vi "Big_LED_control.vi"() -> ()   [LabVIEW 2018]
uses:
  AT lib/AmateurStepperMotor.dll
  <instrlib>/niDMM/nidmm.llb/niDMM Function.ctl
  <instrlib>/niDMM/nidmm.llb/niDMM Resolution in Digits.ctl
  <instrlib>/niDCPower/nidcpower.llb/niDCPower Measurement Type.ctl
  <vilib>/Instr/_visa.llb/VISA Configure Serial Port (Instr).vi
  <instrlib>/niDMM/nidmm.llb/niDMM Configure Measurement Digits.vi
panel:
  in  "Tab Control 2":enum32{"Шаговик и офир", "Служебная область"}(tab)
  in  "milliseconds to wait":u32=1000
  in  "Go To":dbl
  out "Ophir 1 Char":dbl(graph)=7.0
  in  "DecelerationTime, s":dbl
  in  "AccelerationTime, s":dbl
  in  "HoldOn":bool
  in  "Ophir 1 units":string(combo)="1000" caption="Units"
  out "Ophir 1 Over Range":bool caption="Over Range"
  out "Ophir 1 Optical Power":dbl=7.0 caption="Power" format="%#_4g"
  out "Ophir 1 MAX":dbl=7.0200000000000005 caption="MAX" format="%#_5g"
  in  "Ophir 1 Clear":bool caption="Clear"
  in  "StepMultiplicationFactor":dbl=1.0
  in  "StepDivisor":i32(ring)=8 items=["D1"=1, "D2"=2, "D4"=4, "D8"=8, "D16"=16, "D32"=32]
  in  "Speed":dbl=1000.0
  in  "Погнали!":bool
  in  "Стоп GoTo":bool
  out "Готово":bool
  out "Position":dbl
  in  "Ophir 1 Info":u16(ring)=1 caption="Info" items=["Device : JUNO; s/n:903793", "Head : PD300R-3W   ; s/n:779628"]
  in  "new pos":dbl
  in  "set pos":bool
  out "Device Response":string="*\n"
  in  "Ophir 1 usb channel":i16 caption="usb channel"
  out "Ophir 1 dup Visa Session":refnum<visa-resource-name>="USB0::0x0BD3::0x0777::NI-VISA-60004::RAW" caption="dup Visa Session"
  in  "Ophir 1 Baud Rate (3:9600)":i16(ring)=3 caption="Baud Rate (3:9600)" items=["300", "1200", "4800", "9600", "19200", "38400"]
  out "Ophir 1 Real Optical Power":dbl=0.007 format="%.6e"
  in  "Ophir 1 GPIB Address (10)":string="10" caption="GPIB Address (10)"
  in  "Ophir 1 Port Number (default 2)":i16=1 caption="Port Number (default 2)" min=0 max=20
  in  "Ophir 1 Select Communication Protocol":u16(ring) caption="Select Communication Protocol" items=["USB", "RS232", "GPIB"]
  out "Ophir 1 error out":errorcluster caption="error out"
  in  "Ophir 1 error in (no error)":errorcluster caption="error in (no error)"
  in  "Ophir 1 Wait":u32=100 caption="Wait"
  out "IsOpen":bool=TRUE
  out "Ophir 1 Initialization":bool=TRUE caption="Initialization"
  in  "Tab Control":T1(tab)
  in  "POWER":bool
  in  "Стоп":bool
  in  "Resource Name":refnum<k15>="PXI1Slot2" caption="Источник питания"
  in  "Амперметр":refnum<k15>="PXI1Slot4" caption="NI DMM 1"
  in  "V_MB, V":dbl=5.0 caption="voltage level" format="%_6p"
  in  "curlim_V_MB, A":dbl=0.3 caption="current limit" format="%_6p"
  out "curmes_V_MB, A":dbl caption="measurement" format="%_6g"
  out "chart_0":dbl(graph)=-0.001986406197333734 caption="Waveform Chart 5"
  in  "voltlim_I_LED, V":dbl=2.0 caption="current limit" min=0.01 format="%_6p"
  in  "I_LED, A":dbl=0.005 caption="voltage level" format="%_6p"
  out "chart_1":dbl(graph) caption="Waveform Chart 5"
  out "voltmes_I_LED, V":dbl caption="measurement" format="%_6g"
  out "Current Char":dbl(graph)=0.0019995495676994324
  in  "Arduino":refnum<visa-resource-name>="COM14"
  in  "Сегменты":bool[](array[boolean])=[FALSE, FALSE, FALSE, FALSE, FALSE, FALSE, FALSE, FALSE, FALSE, FALSE, FALSE, FALSE, FALSE, FALSE, FALSE, FALSE, FALSE, FALSE]
  in  "Вольтметр":refnum<k15>="PXI1Slot5" caption="NI DMM 1"
  out "Voltage Char":dbl(graph)=nan
  in  "Port Name":string="COM7" caption="Порт шаговика"
  in  "wave_lenght":string="600"
  in  "Промер":bool caption="Промер сегмента"
  in  "NI DMM 1 Voltage Range 4":string(combo)="-1" caption="Range"
  in  "NI DMM 1 units 4":string(combo)="1" caption="Units"
  out "Voltage":dbl=nan format="%_6g"
  in  "NI DMM 1 Current Range 3":string(combo)="1" caption="Range"
  in  "NI DMM 1 units 3":string(combo)="1000" caption="Units"
  out "Current":dbl=0.0019995495676994324 format="%_6g"
  out "Разряд":dbl
  out "+/-":bool
  out "Power off":bool=TRUE
  in  "Command":string="Anode"
  in  "Записать":bool
  out "measure output file refnum":refnum<file>
  out "Voltage, V":dbl=nan caption="Measurement" format="%.5f"
  out "Current, A":dbl=1.9995495676994324e-06 caption="Measurement" format="%.5f"
  out "Тип индикатора":string="Anode"
  out "chart_2":dbl(graph)=4.286668577189643e-07
  in  "V_RES, V":dbl caption="voltage level" format="%_6p"
  out "curmes_V_RES, A":dbl caption="measurement" format="%_6g"
  in  "curlim_V_RES, A":dbl=0.1 caption="current limit" min=0.01 format="%_6p"
  in  "measure path":path=path "D:/NI LabVIEW/MultiOpto/MultiOpto_1.2/Logs/SEL"
  out "Enum":enum16{"Exit", "4", "Промер", "2", "1"}(ring)
  out "№ об-ца":dbl=-1.0
  out "Темп-ра":dbl=-1.0
  out "Сегмент":string
  # "Шаговик"
  # "Офир"
  # "Шаговик"
  # "Офир"
  # "position - это значение абсолютное"
  # "j"
  # "c"
  # "d"
  # "e"
  # "g"
  # "h"
  # "a"
  # "b"
  # "f"
  # "k"
  # "L"
  # "m"
  # "n"
  # "p"
  # "dp"
  # "all"
  # "V_MB 5 В\nогрничение 300 м\n\nV_LED 2,1 В\nограничение 200 м"
  # "единицы мА\nrange 1 А"
  # "1. каждый сегмент включаем по отдельности, резистором постраиваем ток до 10 мА\n2. напряжение V_LED при этом не меняется\n3. в такоом положении промеряем сегменты по отдельности\n4. для промера всего индикатора сразу подстраиваем напряжение при неизменном положении резисторов\n5. ток всех индикаторов = ток одного сегмента (10 мА) * число сегментов (15)\n6. добиваемся этого увеличением V_LED"
  # "единицы В\nrange AUTO"
  # "регклировка суммарного тока через индикатор"
  # "24.063\n\n     I          U\n20 мА  1.3 В\n20 мА  1.4 В\n 7 мА   1.15 В"
  # "24.064\n\n     I          U\n10 мА  2 В\n10 мА  2.15 В\n 7 мА   1.9 В"
  # "автоматизировать подбор напряжения по известному максимальному напряжению и току. ОС по току сегмента"
  # "Р1:  +25°C\nР2:  - 60°C\nР3:  +85°C"
  # "регулировать ток в зависимости от температуры.\nс ростом температуры растет ток.\nпид-регулятор??"
  # "0. ввести номер образца\n1. включить нужный сегмент\n2. ввести его в поле справа\n3. вести температуру в поле слева\n4. нажать кнопку \"промер сегмента\""
  # "\"опрашивать кнопки не чаще, чем раз в секунду. сейчас кликать можно чаще, они загорятся, но ничего не произойдет\""
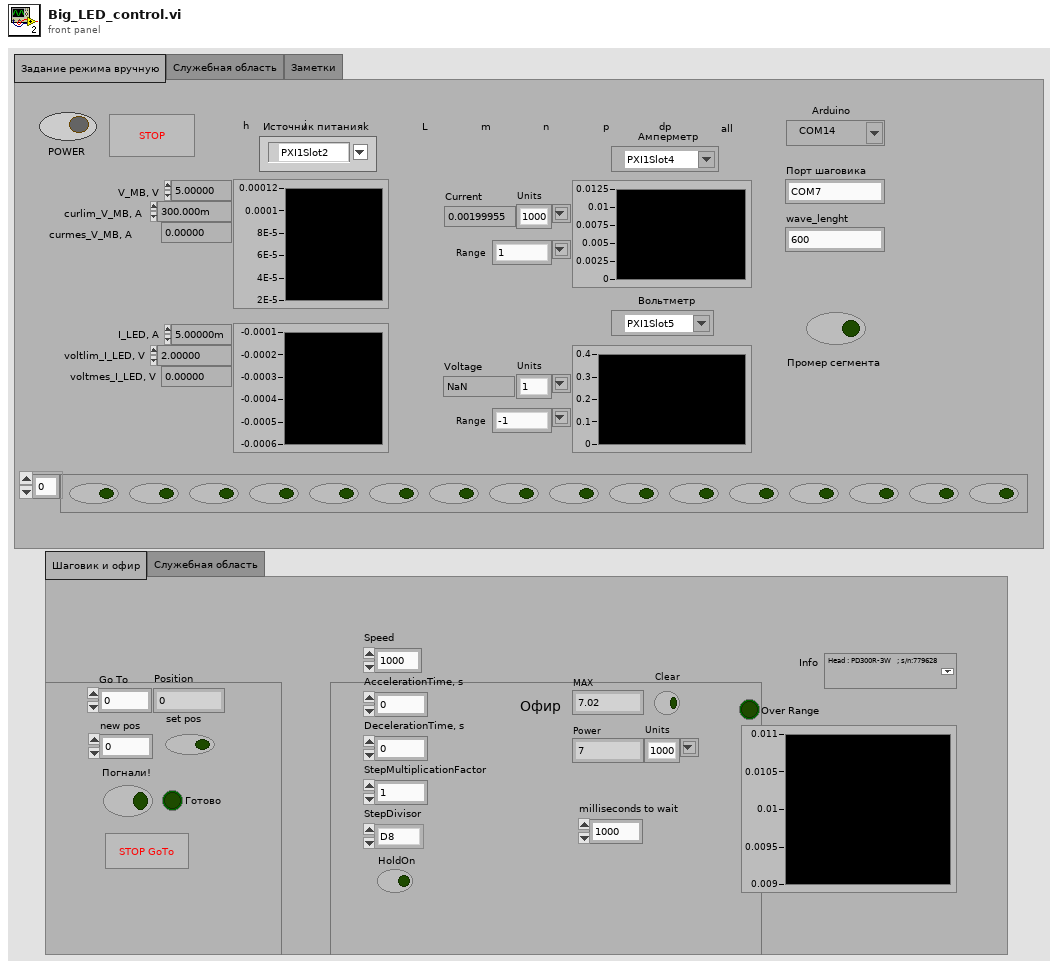
[diagram p1: front panel]
types:
  T1 = enum32{"Задание режима вручную", "Служебная область", "Заметки"}
  T2 = enum16{"open", "replace", "create", "open or create", "replace or create", "replace or create with confirmation"}
  T3 = typedef "niDCPower Measurement Type.ctl" = i32
  T4 = typedef "niDMM Function.ctl" = enum16{"DC Volts", "AC Volts", "DC Current", "AC Current", "2-wire Resistance", "4-wire Resistance", "Diode", "Frequency", "Period", "AC Volts DC Coupled", "Capacitance", "Inductance", "Temperature"}
  T5 = typedef "niDMM Resolution in Digits.ctl" = dbl
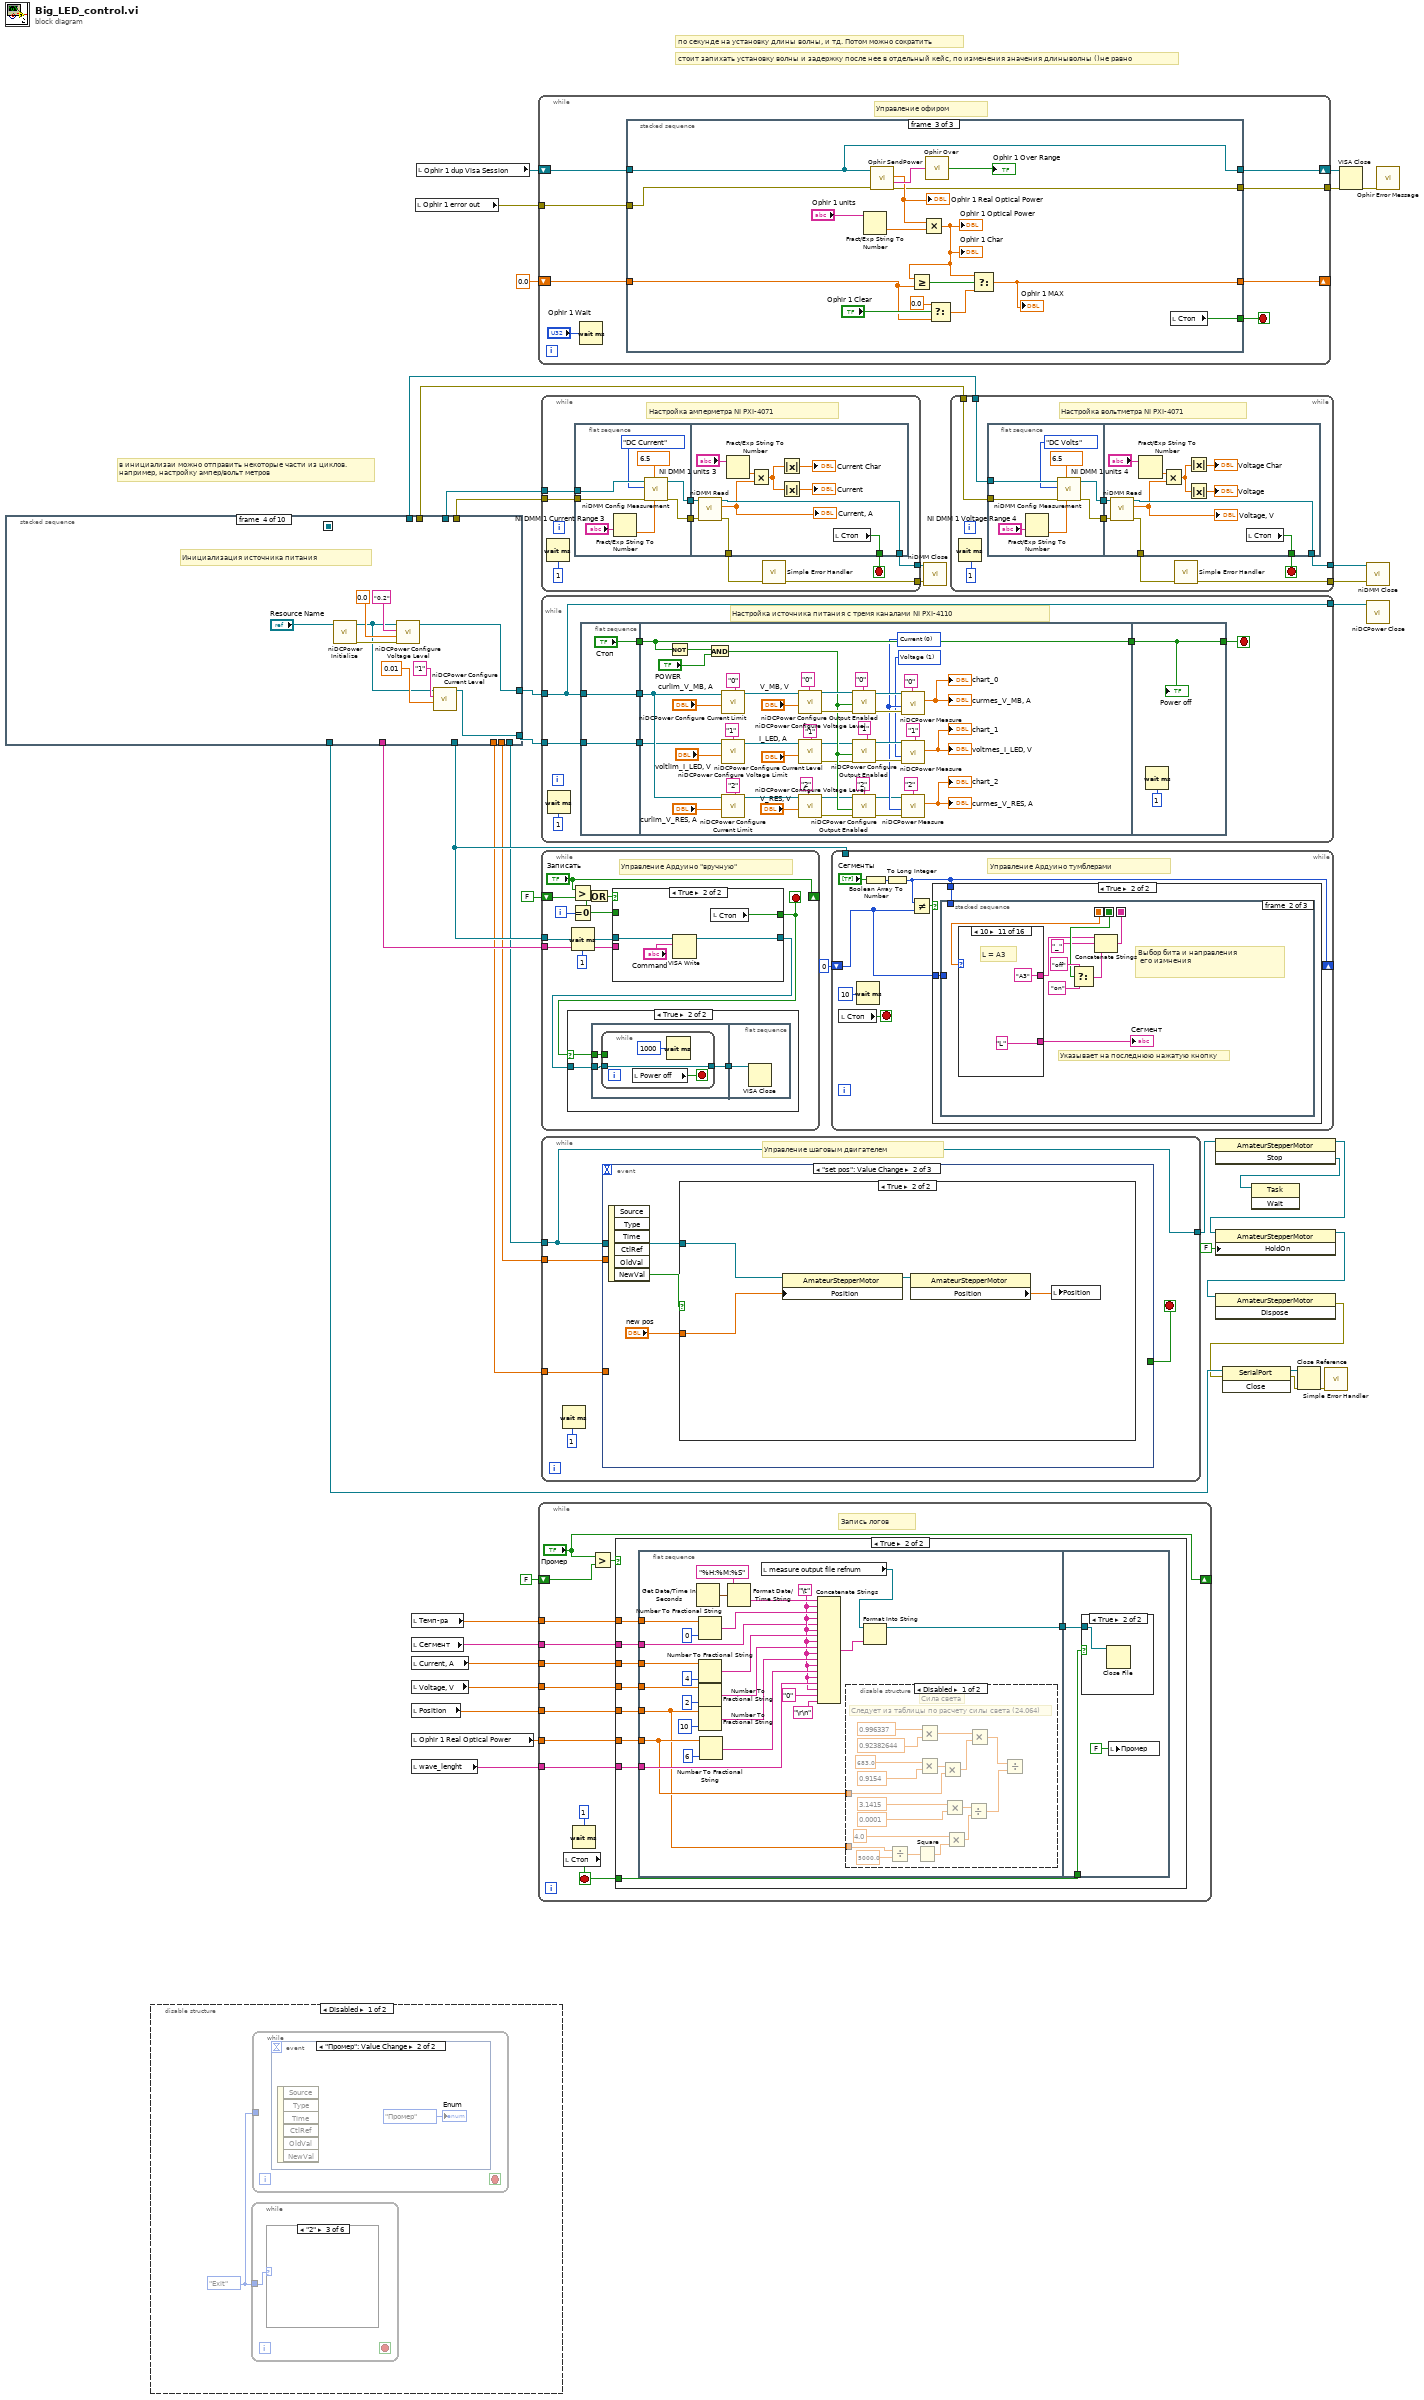
[diagram p0: block diagram]
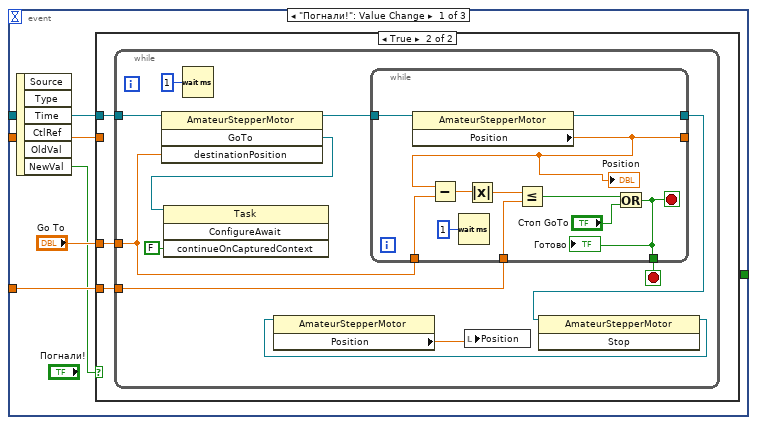
[diagram p2: hidden frame]
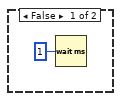
[diagram p3: hidden frame]
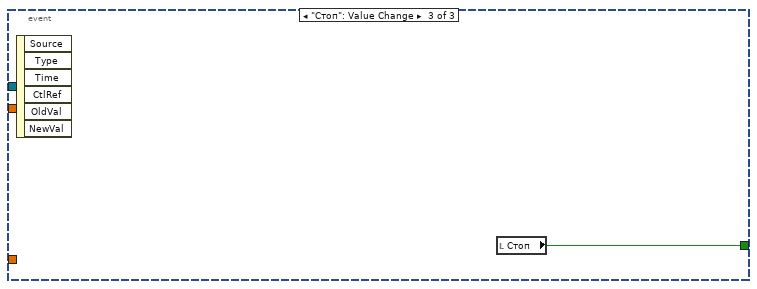
[diagram p5: hidden frame]
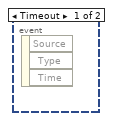
[diagram p11: hidden frame]
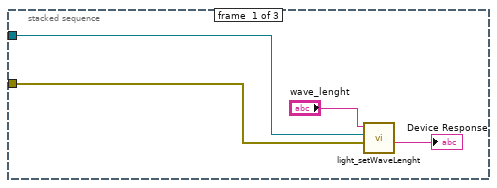
[diagram p16: hidden frame]
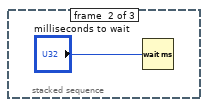
[diagram p17: hidden frame]
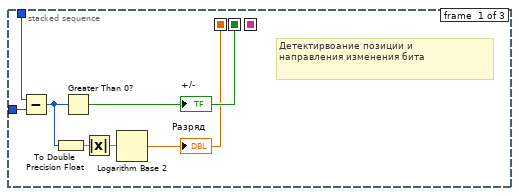
[diagram p19: hidden frame]
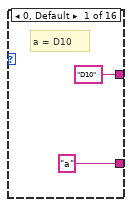
[diagram p20: hidden frame]
diagram:
  # "в инициализаи можно отправить некоторые части из циклов.\nнапример, настройку ампер/вольт метров"
  # "стоит запихать установку волны и задержку после нее в отдельный кейс, по изменения значения длиныволны ()не равно"
  # "по секунде на установку длины волны, и тд. Потом можно сократить"
  n1 = stacked-sequence {
    seq-local: [_ _ _ _ _ _ w95 _ _ _] -> [_ _ _ _ _ _ _ w104 _ _]
    tunnel: [_ _ _ w61 _ _ _ _ _ _] -> w30
    tunnel: [_ w49 _ _ _ _ _ _ _ _] -> w42
    tunnel: [_ w48 _ _ _ _ _ _ _ _] -> w41
    tunnel: [_ _ _ _ w62 _ _ _ _ _] -> w38
    tunnel: [_ _ _ _ _ _ _ _ _ w144] -> w37
    tunnel: [_ _ w52 _ _ _ _ _ _ _] -> w36
    tunnel: [_ _ w51 _ _ _ _ _ _ _] -> w35
    tunnel: [_ _ _ _ _ _ _ w107 _ _] -> w29
    tunnel: [_ _ _ _ _ _ _ w105 _ _] -> w27
    tunnel: [_ _ _ _ _ _ _ w106 _ _] -> w28
    tunnel: [_ _ _ _ _ _ w85 _ _ _] -> w21
    tunnel: [_ _ _ w54 _ _ _ _ _ _] -> w4
    frame #0 {
      w43 = 0.0 ("currentmes_2")
      w44 = FALSE ("Стоп")
      # "Обнуление переменных"
      n2 = local write "POWER"(w44) -> ()
      n3 = local write "Стоп"(w44) -> ()
      n4 = local write "+/-"(w44) -> ()
      n5 = local write "Погнали!"(w44) -> ()
      n6 = local write "Готово"(w44) -> ()
      n7 = local write "Стоп GoTo"(w44) -> ()
      n8 = local write "Go To"(w43) -> ()
      n9 = local write "curmes_V_MB, A"(w43) -> ()
      n10 = local write "curmes_V_RES, A"(w43) -> ()
      n11 = local write "Current"(w43) -> ()
      n12 = local write "Разряд"(w43) -> ()
      n13 = local write "voltmes_I_LED, V"(w43) -> ()
      n14 = local write "Сегменты"(bool[] [FALSE, FALSE, FALSE, FALSE, FALSE, FALSE, FALSE, FALSE, FALSE, FALSE, FALSE, FALSE, FALSE, FALSE, FALSE, FALSE, FALSE, FALSE] ("Сегменты")) -> ()
      n15 = local write "Command"("zero" ("Command 2")) -> ()
    }
    frame #1 {
      # "Инициализация амперметра"
      n16 = call <instrlib>:"niDMM Initialize.vi"("Instrument Descriptor"="Амперметр") -> ("error out"=w49:errorcluster, "instrument handle out"=w48:refnum<k15>)  [unwired: 9 in]
    }
    frame #2 {
      # "Инициализация вольтметра"
      n17 = call <instrlib>:"niDMM Initialize.vi"("Instrument Descriptor"="Вольтметр") -> ("error out"=w51:errorcluster, "instrument handle out"=w52:refnum<k15>)  [unwired: 9 in]
    }
    frame #3 {
      # "Инициализация источника питания"
      n18 = call <instrlib>:"niDCPower Initialize.vi"("resource name"="Resource Name") -> ("error out"=w58:errorcluster, "instrument handle out"=w53:refnum<k15>)  [unwired: 3 in, 6 out]
      n19 = call <instrlib>:"niDCPower Configure Voltage Level.vi"("error in (no error)"=w58, "voltage level"=0.0, "channel name"="0,2", "instrument handle"=w53) -> ("instrument handle out"=w61:refnum<k15>)  [unwired: 6 in, 1 out]
      n20 = call <instrlib>:"niDCPower Configure Current Level.vi"("current level"=0.01, "channel name"="1", "instrument handle"=w53) -> ("instrument handle out"=w54:refnum<k15>)  [unwired: 7 in, 1 out]
    }
    frame #4 {
      # "Инициализация Ардуино"
      n21 = call-poly "VISA Configure Serial Port"("VISA resource name"="Arduino", "baud rate (9600)"=u32 9600) -> ("VISA resource name out"=w62:refnum<visa-resource-name>)  [unwired: 12 in, 1 out]
    }
    frame #5 {
      # "Инициализация офира"
      n22 = call "Ophir InitCom.vi"("GPIB Address (default 10)"="Ophir 1 GPIB Address (10)", "Communication (default USB 0)"="Ophir 1 Select Communication Protocol", "USB Channel number (default 0)"="Ophir 1 usb channel", "Port Number (default 2)"="Ophir 1 Port Number (default 2)", "error in (no error)"="Ophir 1 error in (no error)", "Baud Rate (3:9600)"="Ophir 1 Baud Rate (3:9600)") -> ("dup Visa Session"=w71:refnum<visa-resource-name>, "error out"=w70:errorcluster)  [unwired: 1 out]
      n23 = call "Ophir InstrInfo.vi"("Visa Session"=w71, "error in (no error)"=w70) -> ("dup Visa Session"=w83:refnum<visa-resource-name>, "Instrument Info"=w65:string, "error out"=w81:errorcluster)
      n24 = call "Ophir HeadInfo.vi"("Visa Session"=w83, "error in (no error)"=w81) -> ("error out"=w80:errorcluster, "dup Visa Session"=w82:refnum<visa-resource-name>, "Head Info"=w79:string)  [unwired: 6 out]
      n25 = call "Ophir InfoStrings.vi"("error in (no error)"=w80, "Head Info"=w79, "Instrument Info"=w65) -> ("error out"=w78:errorcluster, "Strings Array"=w77:string[])
      n26 = property on="Ophir 1 Info" class="Ring (strict)"("Strings []"=w77) -> ()  [unwired: 2 in, 2 out]
      n27 = call "Ophir ConfigDevice.vi"("Visa Session"=w82, "Measure Choice (0:Power)"=u16 0, "error in (no error)"=w78) -> ("dup Visa Session"=→"Ophir 1 dup Visa Session":refnum<visa-resource-name>, "OK ?"=→"Ophir 1 Initialization":bool, "error out"=→"Ophir 1 error out":errorcluster)  [unwired: 1 out]
    }
    frame #6 {
      w89 = 100 ("WriteTimeout")
      w94 = 1 items=["None", "One", "Two", "OnePointFive"] ("stopBits")
      w91 = 0 items=["None", "Odd", "Even", "Mark", "Space"] ("parity")
      # "убрали открытие порта. шаговик его и так сам откроет"
      # "Инициализация шаговика ч.1"
      n28 = constructor class="SerialPort"("portName"="Port Name", "baudRate"=57600, "parity"=w91, "dataBits"=8, "stopBits"=w94) -> (reference out=w88:refnum<k24>, error out=w87:errorcluster)  [unwired: 3 in, 6 out]
      n29 = property class="SerialPort"(reference=w88, error in=w87, "WriteTimeout"=w89, "ReadTimeout"=w89) -> (reference out=w85:refnum<k24>)  [unwired: 1 out]
      n30 = constructor class="AmateurStepperMotor"("serialPort"=w85) -> (reference out=w95:refnum<k24>, error out=w86:errorcluster)  [unwired: 3 in, 2 out]
      n31 = flat-sequence {
        tunnel: w86 -> [_]
        tunnel: w85 -> [w97]
        frame #0 {
          n32 = property class="SerialPort"(reference=w97) -> ("IsOpen"=→"IsOpen":bool)  [unwired: 1 in, 2 out]
        }
      }
    }
    frame #7 {
      # "стоит допустить изменение\nтих параметров в цикле, а не только \nпри инициализации"
      # "это те самые 50 шагов за мм"
      # "Инициализация шаговика ч.2"
      n33 = property class="AmateurStepperMotor"(reference=w104, "Speed"="Speed", "StepDivisor"="StepDivisor", "StepMultiplicationFactor"="StepMultiplicationFactor", "AccelerationTime"="AccelerationTime, s", "DecelerationTime"="DecelerationTime, s", "HoldOn"="HoldOn") -> (reference out=w107:refnum<k24>, "Position"=w105:dbl, "PositioningPrecision"=w106:dbl)  [unwired: 1 in, 1 out]
    }
    frame #8 {
      w113 = "\t"
      # "Инициализация логов"
      n34 = local read "№ об-ца"() -> (w109:dbl)
      n35 = Number To Fractional String(number=w109, precision (6)=i16 0) -> (F-format string=w110:string)  [unwired: 2 in]
      n36 = Get Date/Time In Seconds() -> (seconds since 1Jan1904=w131:timestamp)
      n37 = Build Path(base path="measure path", name or relative path=w110) -> (appended path=w127:path)
      n38 = call <vilib>:"Check if File or Folder Exists.vi"("path"=w127) -> ("file or folder exists?"=w128:bool, "dup path"=w129:path)  [unwired: 8 in, 1 out]
      n39 = Format Date/Time String(time format string (%c)="MES %d %m %y %H.%M.%S", seconds (now)=w131) -> (date/time string=w132:string)  [unwired: 1 in]
      n40 = case shown="False" w128 {
        tunnel: w129 -> [w140 w141]
        tunnel: [w139 w141] -> w130
        frame False {
          n41 = Create Folder(path (use dialog)=w140) -> (created path=w139:path)  [unwired: 2 in, 2 out]
        }
        frame True {
        }
      }
      n42 = Concatenate Strings(w132, ".xls" ("string")) -> (w133:string)
      n43 = Build Path(base path=w130, name or relative path=w133) -> (appended path=w134:path)
      n44 = Open/Create/Replace File(file path (use dialog)=w134, operation (0:open)=T2."open or create", access (0:read/write)=enum16{"read/write", "read-only", "write-only"}."read/write") -> (refnum out=w135:refnum<file>)  [unwired: 3 in, 2 out]
      n45 = Set File Position(refnum=w135, from (0:start)=enum16{"start", "end", "current"}."end") -> (refnum out=w137:refnum<file>)  [unwired: 2 in, 1 out]
      n46 = Format Into String(initial string=w137, "Time" ("string"), w113, "Temperature, C" ("string"), w113, "Segment" ("string"), w113, "Current, mA" ("string"), w113, "Voltage, V" ("input 7"), w113, "Distance, m" ("string"), w113, "Power, W " ("string"), w113, "Wavelenght, nm" ("input 17"), w113, "Candlepower, kd" ("string"), "\r\n") -> (resulting string=→"measure output file refnum":refnum<file>)  [unwired: 2 in, 1 out]
    }
    frame #9 {
      # "Begin VI: ОК или ОА?"
      n47 = call "Begin.vi"() -> ("Темп-ра"=→"Темп-ра":dbl, "№ об-ца"=→"№ об-ца":dbl, "String"=w144:string)  [unwired: 6 in]
      "Тип индикатора" <- w144
      n48 = local write "Command"(w144) -> ()
    }
  }
  n49 = disable-structure shown="Disabled" {
    frame Disabled {
      w145 = enum16{"Exit", "4", "Промер", "2", "1"}."Exit"
      n50 = while {
        tunnel: w145 -> [w146]
        stop <- _ stop-if-true
        n51 = case shown="\"2\"" w146 {
          frame "Exit", Default {
          }
          frame "4" {
          }
          frame "2" {
          }
          frame "2" {
          }
          frame "1" {
          }
          frame "Промер" {
          }
        }
      }
      n52 = while {
        tunnel: w145 -> [_]
        stop <- _ stop-if-true
        n53 = event shown="[1] \"Промер\": Value Change" {
          selector: _ -> [_ _]
          dyn-events: _ -> [_ _]
          timeout: _ -> [_ _]
          event Timeout {
            n54 = event-data() -> ()  [unwired: 1 in, 3 out]
          }
          event "Промер": Value Change {
            n55 = event-data() -> ()  [unwired: 1 in, 6 out]
            "Enum" <- enum16{"Exit", "4", "Промер", "2", "1"}."Промер" ("Enum")
          }
        }
      }
    }
    frame Enabled {
    }
  }
  n56 = local read "Темп-ра"() -> (w2:dbl)
  n57 = local read "Сегмент"() -> (w1:string)
  n58 = local read "Current, A"() -> (w20:dbl)
  n59 = local read "Voltage, V"() -> (w19:dbl)
  n60 = local read "Position"() -> (w18:dbl)
  n61 = local read "Ophir 1 Real Optical Power"() -> (w17:dbl)
  n62 = local read "wave_lenght"() -> (w16:string)
  n63 = local read "Ophir 1 error out"() -> (w25:errorcluster)
  n64 = local read "Ophir 1 dup Visa Session"() -> (w26:refnum<visa-resource-name>)
  n65 = while {
    tunnel: w20 -> [w159]
    tunnel: w19 -> [w158]
    tunnel: w18 -> [w157]
    tunnel: w17 -> [w156]
    tunnel: w16 -> [w155]
    shift-right: ["Промер"] -> _
    shift-left: FALSE ("Промер сегмента") -> [w152]
    tunnel: w2 -> [w149]
    tunnel: w1 -> [w148]
    stop <- w150 stop-if-true
    # "Запиcь логов"
    n66 = local read "Стоп"() -> (w150:bool)
    n67 = Wait (ms)(milliseconds to wait=u32 1) -> ()  [unwired: 1 out]
    n68 = Greater?(x="Промер", y=w152) -> (0:w153:bool)
    n69 = case shown="True" w153 {
      tunnel: w159 -> [_ w168]
      tunnel: w158 -> [_ w167]
      tunnel: w157 -> [_ w164]
      tunnel: w156 -> [_ w165]
      tunnel: w155 -> [_ w166]
      tunnel: w150 -> [_ w162]
      tunnel: w149 -> [_ w161]
      tunnel: w148 -> [_ w160]
      frame False {
      }
      frame True {
        n70 = flat-sequence {
          tunnel: w168 -> [w186]
          tunnel: w167 -> [w185]
          tunnel: w166 -> [w183]
          tunnel: w165 -> [w182]
          tunnel: w164 -> [w181]
          tunnel: [w176] -> w163
          tunnel: w161 -> [w175]
          tunnel: w160 -> [w169]
          tunnel: w163 -> [w216]
          tunnel: w162 -> [w215]
          frame #0 {
            w171 = "\t"
            n71 = Get Date/Time In Seconds() -> (seconds since 1Jan1904=w194:timestamp)
            n72 = Number To Fractional String(number=w175, precision (6)=i16 0) -> (F-format string=w173:string)  [unwired: 2 in]
            n73 = Number To Fractional String(number=w186, precision (6)=i16 4) -> (F-format string=w189:string)  [unwired: 2 in]
            n74 = Number To Fractional String(number=w185, precision (6)=i16 2) -> (F-format string=w188:string)  [unwired: 2 in]
            n75 = Number To Fractional String(number=w181, precision (6)=i16 10) -> (F-format string=w187:string)  [unwired: 2 in]
            n76 = Number To Fractional String(number=w182, precision (6)=i16 6) -> (F-format string=w184:string)  [unwired: 2 in]
            n77 = Format Date/Time String(time format string (%c)="%H:%M:%S", seconds (now)=w194) -> (date/time string=w192:string)  [unwired: 1 in]
            n78 = local read "measure output file refnum"() -> (w190:refnum<file>)
            n79 = Concatenate Strings(w192, w171, w173, w171, w169, w171, w189, w171, w188, w171, w187, w171, w184, w171, w183, w171, "0" ("string"), "\r\n") -> (w191:string)
            n80 = disable-structure shown="Disabled" {
              disable-tunnel: w182 -> [w206 _]
              disable-tunnel: w181 -> [w196 _]
              frame Disabled {
                # "Сила света"
                # "Следует из таблицы по расчету силы света (24.064)"
                n81 = Divide(x=w196, y=5000.0) -> (x/y=w198:dbl)
                n82 = Square(x=w198) -> (x^2=w197:dbl)
                n83 = Multiply(x=0.996337, y=0.92382644) -> (x*y=w211:dbl)
                n84 = Multiply(x=683.0, y=0.9154) -> (x*y=w207:dbl)
                n85 = Multiply(x=w207, y=w206) -> (x*y=w205:dbl)
                n86 = Multiply(x=3.1415, y=0.0001) -> (x*y=w201:dbl)
                n87 = Multiply(x=4.0, y=w197) -> (x*y=w200:dbl)
                n88 = Divide(x=w201, y=w200) -> (x/y=w202:dbl)
                n89 = Multiply(x=w211, y=w205) -> (x*y=w210:dbl)
                n90 = Divide(x=w210, y=w202) -> ()  [unwired: 1 out]
              }
              frame Enabled {
              }
            }
            n91 = Format Into String(initial string=w190, w191) -> (resulting string=w176:refnum<file>)  [unwired: 2 in, 1 out]
          }
          frame #1 {
            n92 = case shown="True" w215 {
              tunnel: w216 -> [_ w217]
              frame False {
              }
              frame True {
                n93 = Close File(refnum=w217) -> ()  [unwired: 1 in, 2 out]
              }
            }
            n94 = local write "Промер"(FALSE ("Промер")) -> ()
          }
        }
      }
    }
  }
  n95 = while {
    tunnel: w25 -> [w224]
    shift-right: [w220] -> _
    shift-left: 0.0 ("t") -> [w223]
    shift-right: [w221] -> w14
    shift-left: w26 -> [w225]
    tunnel: [w219] -> w13
    stop <- w218 stop-if-true
    # "Управление офиром"
    n96 = Wait (ms)(milliseconds to wait="Ophir 1 Wait") -> ()  [unwired: 1 out]
    n97 = stacked-sequence {
      tunnel: w225 -> [w229 _ w232]
      tunnel: w224 -> [w228 _ w234]
      tunnel: w223 -> [_ _ w235]
      tunnel: [_ _ w232] -> w221
      tunnel: [_ _ w236] -> w220
      tunnel: [_ _ w233] -> w219
      tunnel: [_ _ w231] -> w218
      frame #0 {
        n98 = call "light_setWaveLenght.vi"("error in (no error)"=w228, "Visa Session"=w229, "wave_lenght"="wave_lenght") -> ("Device Response"=→"Device Response":string)  [unwired: 6 in, 2 out]
      }
      frame #1 {
        n99 = Wait (ms)(milliseconds to wait="milliseconds to wait") -> ()  [unwired: 1 out]
      }
      frame #2 {
        n100 = Fract/Exp String To Number(string="Ophir 1 units") -> (number=w239:dbl)  [unwired: 3 in, 1 out]
        n101 = call "Ophir SendPower.vi"("Visa Session"=w232, "error in (no error)"=w234) -> ("Value Number"=w238:dbl, "Value String"=w245:string, "error out"=w233:errorcluster)  [unwired: 1 out]
        "Ophir 1 Real Optical Power" <- w238
        n102 = Multiply(x=w238, y=w239) -> (x*y=w242:dbl)
        "Ophir 1 Char" <- w242
        "Ophir 1 Optical Power" <- w242
        n103 = Greater Or Equal?(x=w242, y=w235) -> (x >= y?=w243:bool)
        n104 = call "Ophir Over.vi"("Value String"=w245) -> ("Overrange"=→"Ophir 1 Over Range":bool)
        n105 = Select(t=0.0, s="Ophir 1 Clear", f=w235) -> (s? t:f=w241:dbl)
        n106 = Select(t=w242, s=w243, f=w241) -> (s? t:f=w236:dbl)
        "Ophir 1 MAX" <- w236
        n107 = local read "Стоп"() -> (w231:bool)
      }
    }
  }
  n108 = while {
    tunnel: w30 -> [w251]
    tunnel: [w251] -> w39
    tunnel: w4 -> [w248]
    stop <- w247 stop-if-true
    # "Настройка источника питания с тремя каналами NI PXI-4110"
    n109 = Wait (ms)(milliseconds to wait=u32 1) -> ()  [unwired: 1 out]
    n110 = flat-sequence {
      tunnel: w251 -> [w257]
      tunnel: [w257] -> w253
      tunnel: ["Стоп"] -> w252
      tunnel: [w255] -> w249
      tunnel: w248 -> [w255]
      tunnel: w253 -> [w291]
      tunnel: w252 -> [w301]
      tunnel: [w301] -> w250
      tunnel: w249 -> [w285]
      tunnel: [w303] -> w247
      tunnel: w250 -> [w303]
      frame #0 {
      }
      frame #1 {
        w278 = T3 1 items=["Current", "Voltage"] ("measurement type")
        w290 = T3 0 items=["Current", "Voltage"] ("measurement type")
        n111 = Not(x=w301) -> (.not. x?=w300:bool)
        n112 = And(x=w300, y="POWER") -> (x .and. y?=w288:bool)
        n113 = call <instrlib>:"niDCPower Configure Current Limit.vi"("current limit"="curlim_V_MB, A", "channel name"="0", "instrument handle"=w291) -> ("instrument handle out"=w276:refnum<k15>)  [unwired: 7 in, 1 out]
        n114 = call <instrlib>:"niDCPower Configure Voltage Limit.vi"("voltage limit"="voltlim_I_LED, V", "channel name"="1", "instrument handle"=w285) -> ("instrument handle out"=w282:refnum<k15>)  [unwired: 7 in, 1 out]
        n115 = call <instrlib>:"niDCPower Configure Current Limit.vi"("current limit"="curlim_V_RES, A", "channel name"="2", "instrument handle"=w291) -> ("instrument handle out"=w267:refnum<k15>)  [unwired: 7 in, 1 out]
        n116 = call <instrlib>:"niDCPower Configure Voltage Level.vi"("voltage level"="V_MB, V", "channel name"="0", "instrument handle"=w276) -> ("error out"=w296:errorcluster, "instrument handle out"=w295:refnum<k15>)  [unwired: 7 in]
        n117 = call <instrlib>:"niDCPower Configure Current Level.vi"("current level"="I_LED, A", "channel name"="1", "instrument handle"=w282) -> ("error out"=w280:errorcluster, "instrument handle out"=w283:refnum<k15>)  [unwired: 7 in]
        n118 = call <instrlib>:"niDCPower Configure Voltage Level.vi"("voltage level"="V_RES, V", "channel name"="2", "instrument handle"=w267) -> ("error out"=w269:errorcluster, "instrument handle out"=w268:refnum<k15>)  [unwired: 7 in]
        n119 = call <instrlib>:"niDCPower Configure Output Enabled.vi"("error in (no error)"=w296, "output enabled"=w288, "channel name"="0", "instrument handle"=w295) -> ("error out"=w293:errorcluster, "instrument handle out"=w294:refnum<k15>)  [unwired: 6 in]
        n120 = call <instrlib>:"niDCPower Configure Output Enabled.vi"("error in (no error)"=w280, "output enabled"=w288, "channel name"="1", "instrument handle"=w283) -> ("error out"=w298:errorcluster, "instrument handle out"=w297:refnum<k15>)  [unwired: 6 in]
        n121 = call <instrlib>:"niDCPower Configure Output Enabled.vi"("error in (no error)"=w269, "output enabled"=w288, "channel name"="2", "instrument handle"=w268) -> ("error out"=w265:errorcluster, "instrument handle out"=w264:refnum<k15>)  [unwired: 6 in]
        n122 = call <instrlib>:"niDCPower Measure.vi"("error in (no error)"=w293, "measurement type"=w290, "channel name"="0", "instrument handle"=w294) -> ("measurement"=→"curmes_V_MB, A" →"chart_0":dbl)  [unwired: 5 in, 2 out]
        n123 = call <instrlib>:"niDCPower Measure.vi"("error in (no error)"=w298, "measurement type"=w278, "channel name"="1", "instrument handle"=w297) -> ("measurement"=→"chart_1" →"voltmes_I_LED, V":dbl)  [unwired: 5 in, 2 out]
        n124 = call <instrlib>:"niDCPower Measure.vi"("error in (no error)"=w265, "measurement type"=w290, "channel name"="2", "instrument handle"=w264) -> ("measurement"=→"curmes_V_RES, A" →"chart_2":dbl)  [unwired: 5 in, 2 out]
      }
      frame #2 {
        n125 = Wait (ms)(milliseconds to wait=u32 1) -> ()  [unwired: 1 out]
        "Power off" <- w303
      }
    }
  }
  n126 = while {
    tunnel: w38 -> [w311]
    shift-right: ["Записать"] -> _
    shift-left: FALSE ("Записать") -> [w313]
    tunnel: w37 -> [w309]
    i -> [w310]
    stop <- w304 stop-if-true
    # "Управление Ардуино \"вручную\""
    n127 = Greater?(x="Записать", y=w313) -> (0:w307:bool)
    n128 = Equal To 0?(x=w310) -> (x = 0?=w306:bool)
    n129 = Wait (ms)(milliseconds to wait=u32 1) -> ()  [unwired: 1 out]
    n130 = Or(x=w307, y=w306) -> (x .or. y?=w308:bool)
    n131 = case shown="True" w308 {
      tunnel: w311 -> [w325 w330]
      tunnel: [w326 w329] -> w304
      tunnel: w309 -> [_ _]
      tunnel: w306 -> [_ _]
      tunnel: [w325 w327] -> w305
      frame False {
        n132 = local read "Стоп"() -> (w326:bool)
      }
      frame True {
        n133 = VISA Write(VISA resource name=w330, write buffer="Command") -> (VISA resource name out=w327:refnum<visa-resource-name>)  [unwired: 1 in, 2 out]
        n134 = local read "Стоп"() -> (w329:bool)
      }
    }
    n135 = case shown="True" w304 {
      selector: w304 -> [_ w315]
      tunnel: w305 -> [_ w317]
      frame False {
      }
      frame True {
        n136 = flat-sequence {
          tunnel: w317 -> [w320]
          tunnel: [w319] -> w316
          tunnel: w315 -> [w318]
          tunnel: w316 -> [w324]
          frame #0 {
            n137 = while {
              tunnel: w320 -> [w323]
              tunnel: [w323] -> w319
              tunnel: w318 -> [_]
              stop <- w321 stop-if-true
              n138 = local read "Power off"() -> (w321:bool)
              n139 = Wait (ms)(milliseconds to wait=u32 1000) -> ()  [unwired: 1 out]
            }
          }
          frame #1 {
            n140 = VISA Close(VISA resource name=w324) -> ()  [unwired: 1 in, 1 out]
          }
        }
      }
    }
  }
  n141 = while {
    tunnel: [w337] -> w31
    tunnel: w41 -> [w335]
    tunnel: w42 -> [w334]
    tunnel: [w331] -> w32
    stop <- w333 stop-if-true
    # "Настройка амперметра NI PXI-4071"
    n142 = Wait (ms)(milliseconds to wait=u32 1) -> ()  [unwired: 1 out]
    n143 = flat-sequence {
      tunnel: [w344] -> w339
      tunnel: w335 -> [w342]
      tunnel: w334 -> [w346]
      tunnel: [w343] -> w338
      tunnel: w339 -> [w355]
      tunnel: w338 -> [w358]
      tunnel: [w354] -> w333
      tunnel: [w353] -> w331
      tunnel: [w352] -> w332
      frame #0 {
        w340 = T5 6.5 items=["3 1/2"=3.5, "4 1/2"=4.5, "5 1/2"=5.5, "6 1/2"=6.5, "7 1/2"=7.5] ("Resolution in Digits")
        n144 = Fract/Exp String To Number(string="NI DMM 1 Current Range 3") -> (number=w345:dbl)  [unwired: 3 in, 1 out]
        n145 = call-poly <instrlib>:"niDMM Config Measurement.vi"("Range"=w345, "Resolution in Digits"=w340, "error in (no error)"=w346, "Function"=niDMM_Function."DC Current" ("Measurement Type"), "instrument handle"=w342) -> ("error out"=w343:errorcluster, "instrument handle out"=w344:refnum<k15>)  [unwired: 5 in]
      }
      frame #1 {
        n146 = call <instrlib>:"niDMM Read.vi"("error in (no error)"=w358, "instrument handle"=w355) -> ("error out"=w352:errorcluster, "Measurement"=w348:dbl, "instrument handle out"=w353:refnum<k15>)  [unwired: 7 in]
        "Current, A" <- w348
        n147 = Fract/Exp String To Number(string="NI DMM 1 units 3") -> (number=w356:dbl)  [unwired: 3 in, 1 out]
        n148 = Multiply(x=w356, y=w348) -> (x*y=w349:dbl)
        n149 = Absolute Value(x=w349) -> (abs(x)=→"Current Char":dbl)
        n150 = Absolute Value(x=w349) -> (abs(x)=→"Current":dbl)
        n151 = local read "Стоп"() -> (w354:bool)
      }
    }
    n152 = call <vilib>:"Simple Error Handler.vi"("error in (no error)"=w332) -> ("error out"=w337:errorcluster)  [unwired: 1 in, 7 out]
  }
  n153 = while {
    tunnel: w29 -> [w360]
    tunnel: w28 -> [w362]
    tunnel: [w360] -> w3
    tunnel: w27 -> [w363]
    stop <- w359 stop-if-true
    # "Управление шаговым двигателем"
    n154 = Wait (ms)(milliseconds to wait=u32 1) -> ()  [unwired: 1 out]
    n155 = event shown="[1] \"set pos\": Value Change" {
      selector: _ -> [_ _ _]
      dyn-events: _ -> [_ _ _]
      timeout: _ -> [_ _ _]
      tunnel: w360 -> [w368 w396 _]
      tunnel: w363 -> [w367 _ _]
      tunnel: w362 -> [w366 _ _]
      tunnel: [_ _ w402] -> w359
      event "Погнали!": Value Change {
        n156 = event-data() -> ("NewVal"=w364:bool)  [unwired: 1 in, 5 out]
        n157 = case shown="True" w364 {
          tunnel: "Go To" -> [_ w372]
          tunnel: w368 -> [_ w371]
          tunnel: w367 -> [_ _]
          tunnel: w366 -> [_ w370]
          frame False {
            n158 = Wait (ms)(milliseconds to wait=u32 1) -> ()  [unwired: 1 out]
          }
          frame True {
            n159 = while {
              tunnel: w372 -> [w379]
              tunnel: w371 -> [w380]
              tunnel: w370 -> [w382]
              stop <- w383 stop-if-true
              n160 = invoke class="AmateurStepperMotor" method="GoTo"(reference=w380, "destinationPosition"=w379) -> (reference out=w375:refnum<k24>, "GoTo"=w378:refnum<k24>)  [unwired: 2 in, 2 out]
              n161 = invoke class="Task" method="ConfigureAwait"(reference=w378, "continueOnCapturedContext"=FALSE) -> ()  [unwired: 2 in, 4 out]
              n162 = Wait (ms)(milliseconds to wait=u32 1) -> ()  [unwired: 1 out]
              n163 = while {
                tunnel: [w384] -> _
                tunnel: [w386] -> w376
                tunnel: [w388] -> w383
                tunnel: w379 -> [w393]
                tunnel: w382 -> [w391]
                tunnel: w375 -> [w385]
                stop <- w388 stop-if-true
                n164 = property class="AmateurStepperMotor"(reference=w385) -> (reference out=w386:refnum<k24>, "Position"=w384:dbl)  [unwired: 1 in, 1 out]
                "Position" <- w384
                n165 = Subtract(x=w384, y=w393) -> (x-y=w394:dbl)
                n166 = Wait (ms)(milliseconds to wait=u32 1) -> ()  [unwired: 1 out]
                n167 = Absolute Value(x=w394) -> (abs(x)=w392:dbl)
                n168 = Less Or Equal?(x=w392, y=w391) -> (x <= y?=w390:bool)
                n169 = Or(x=w390, y="Стоп GoTo") -> (x .or. y?=w388:bool)
                "Готово" <- w388
              }
              n170 = invoke class="AmateurStepperMotor" method="Stop"(reference=w376) -> (reference out=w374:refnum<k24>)  [unwired: 2 in, 2 out]
              n171 = property class="AmateurStepperMotor"(reference=w374) -> ("Position"=w373:dbl)  [unwired: 1 in, 2 out]
              n172 = local write "Position"(w373) -> ()
            }
          }
        }
      }
      event "set pos": Value Change {
        n173 = event-data() -> ("NewVal"=w397:bool)  [unwired: 1 in, 5 out]
        n174 = case shown="True" w397 {
          tunnel: w396 -> [_ w401]
          tunnel: "new pos" -> [_ w400]
          frame False {
          }
          frame True {
            n175 = property class="AmateurStepperMotor"(reference=w401, "Position"=w400) -> (reference out=w399:refnum<k24>)  [unwired: 1 in, 1 out]
            n176 = property class="AmateurStepperMotor"(reference=w399) -> ("Position"=w398:dbl)  [unwired: 1 in, 2 out]
            n177 = local write "Position"(w398) -> ()
          }
        }
      }
      event "Стоп": Value Change {
        n178 = event-data() -> ()  [unwired: 1 in, 6 out]
        n179 = local read "Стоп"() -> (w402:bool)
      }
    }
  }
  n180 = while {
    shift-right: [w405] -> _
    shift-left: 0 -> [w406]
    tunnel: w38 -> [_]
    stop <- w409 stop-if-true
    # "Управление Ардуино тумблерами"
    n181 = local read "Стоп"() -> (w409:bool)
    n182 = Wait (ms)(milliseconds to wait=u32 10 ("millisecond timer value")) -> ()  [unwired: 1 out]
    n183 = Boolean Array To Number(Boolean array="Сегменты") -> (number=w404:u32)
    n184 = To Long Integer(number=w404) -> (32bit integer=w405:i32)
    n185 = Not Equal?(x=w405, y=w406) -> (x != y?=w407:bool)
    n186 = case shown="True" w407 {
      tunnel: w405 -> [_ w410]
      tunnel: w406 -> [_ w411]
      frame False {
      }
      frame True {
        n187 = stacked-sequence {
          seq-local: [w414 _ _] -> [_ w425 _]
          seq-local: [w412 _ _] -> [_ w420 _]
          seq-local: [_ w421 _] -> [_ _ w461]
          tunnel: w410 -> [w416 _ _]
          tunnel: w411 -> [w415 _ _]
          frame #0 {
            # "Детектирвоание позиции и\nнаправления изменения бита"
            n188 = Subtract(x=w416, y=w415) -> (x-y=w417:i32)
            n189 = To Double Precision Float(number=w417) -> (double precision float=w418:dbl)
            n190 = Greater Than 0?(x=w417) -> (x > 0?=w414:bool)
            "+/-" <- w414
            n191 = Absolute Value(x=w418) -> (abs(x)=w413:dbl)
            n192 = Logarithm Base 2(1:w413) -> (0:w412:dbl)
            "Разряд" <- w412
          }
          frame #1 {
            # "Указывает на последнюю нажатую кнопку"
            # "Выбор бита и направления\n его измнения"
            n193 = case shown="10" w420 {
              tunnel: ["D10" "D9" "D5" "D8" "D11" "D12" "A1" "D4" "A5" "A4" "A3" "A2" "A0" "D13" "D3" "All"] -> w423
              tunnel: ["a" "b" "c" "d" "e" "f" "g" "h" "j" "k" "L" "m" "n" "p" "dp" "All"] -> w419
              frame 0, Default {
                # "a = D10"
              }
              frame 1 {
                # "b = D9"
              }
              frame 2 {
                # "c = D5"
              }
              frame 3 {
                # "d = D8"
              }
              frame 4 {
                # "e = D11"
              }
              frame 5 {
                # "f = D12"
              }
              frame 6 {
                # "g = A1"
              }
              frame 7 {
                # "h = D4"
              }
              frame 8 {
                # "j = A5"
              }
              frame 9 {
                # "k = A4"
              }
              frame 10 {
                # "L = A3"
              }
              frame 11 {
                # "m = A2"
              }
              frame 12 {
                # "n = A0"
              }
              frame 13 {
                # "p = D13"
              }
              frame 14 {
                # "dp = D3"
              }
              frame 15 {
              }
            }
            "Сегмент" <- w419
            n194 = Select(t="off", s=w425, f="on") -> (s? t:f=w422:string)
            n195 = Concatenate Strings(w423, "_" ("string"), w422) -> (w421:string)
          }
          frame #2 {
            # "Передача команды в Ардуино"
            n196 = Equal?(x=w461, y="All_off") -> (x = y?=w464:bool)
            n197 = Equal?(x=w461, y="All_on") -> (x = y?=w462:bool)
            n198 = case shown="True" w464 {
              frame False {
              }
              frame True {
                n199 = local write "Сегменты"(bool[] [TRUE, TRUE, TRUE, TRUE, TRUE, TRUE, TRUE, TRUE, TRUE, TRUE, TRUE, TRUE, TRUE, TRUE, TRUE, TRUE] ("Сегменты")) -> ()
              }
            }
            n200 = case shown="True" w462 {
              frame False {
              }
              frame True {
                n201 = local write "Сегменты"(bool[] [FALSE, FALSE, FALSE, FALSE, FALSE, FALSE, FALSE, FALSE, FALSE, FALSE, FALSE, FALSE, FALSE, FALSE, FALSE, FALSE] ("Сегменты")) -> ()
              }
            }
            n202 = stacked-sequence {
              tunnel: w461 -> [w467 _ _]
              frame #0 {
                n203 = local write "Command"(w467) -> ()
              }
              frame #1 {
                n204 = local write "Записать"(TRUE ("Записать")) -> ()
                n205 = Wait (ms)(milliseconds to wait=u32 1000) -> ()  [unwired: 1 out]
              }
              frame #2 {
                n206 = local write "Записать"(FALSE ("Записать")) -> ()
                n207 = Wait (ms)(milliseconds to wait=u32 1000) -> ()  [unwired: 1 out]
              }
            }
          }
        }
      }
    }
  }
  n208 = call <instrlib>:"niDMM Close.vi"("error in (no error)"=w31, "instrument handle"=w32) -> ()  [unwired: 9 in, 1 out]
  n209 = while {
    tunnel: [w478] -> w33
    tunnel: w36 -> [w476]
    tunnel: w35 -> [w475]
    tunnel: [w472] -> w34
    stop <- w474 stop-if-true
    # "Настройка вольтметра NI PXI-4071"
    n210 = Wait (ms)(milliseconds to wait=u32 1) -> ()  [unwired: 1 out]
    n211 = flat-sequence {
      tunnel: [w485] -> w480
      tunnel: w476 -> [w483]
      tunnel: w475 -> [w487]
      tunnel: [w484] -> w479
      tunnel: w480 -> [w496]
      tunnel: w479 -> [w499]
      tunnel: [w495] -> w474
      tunnel: [w494] -> w472
      tunnel: [w493] -> w473
      frame #0 {
        w481 = T5 6.5 items=["3 1/2"=3.5, "4 1/2"=4.5, "5 1/2"=5.5, "6 1/2"=6.5, "7 1/2"=7.5] ("Resolution in Digits")
        n212 = Fract/Exp String To Number(string="NI DMM 1 Voltage Range 4") -> (number=w486:dbl)  [unwired: 3 in, 1 out]
        n213 = call-poly <instrlib>:"niDMM Config Measurement.vi"("Range"=w486, "Resolution in Digits"=w481, "error in (no error)"=w487, "Function"=niDMM_Function."DC Volts" ("Measurement Type"), "instrument handle"=w483) -> ("error out"=w484:errorcluster, "instrument handle out"=w485:refnum<k15>)  [unwired: 5 in]
      }
      frame #1 {
        n214 = call <instrlib>:"niDMM Read.vi"("error in (no error)"=w499, "instrument handle"=w496) -> ("error out"=w493:errorcluster, "Measurement"=w491:dbl, "instrument handle out"=w494:refnum<k15>)  [unwired: 7 in]
        "Voltage, V" <- w491
        n215 = Fract/Exp String To Number(string="NI DMM 1 units 4") -> (number=w497:dbl)  [unwired: 3 in, 1 out]
        n216 = Multiply(x=w497, y=w491) -> (x*y=w489:dbl)
        n217 = Absolute Value(x=w489) -> (abs(x)=→"Voltage Char":dbl)
        n218 = Absolute Value(x=w489) -> (abs(x)=→"Voltage":dbl)
        n219 = local read "Стоп"() -> (w495:bool)
      }
    }
    n220 = call <vilib>:"Simple Error Handler.vi"("error in (no error)"=w473) -> ("error out"=w478:errorcluster)  [unwired: 1 in, 7 out]
  }
  n221 = invoke class="AmateurStepperMotor" method="Stop"(reference=w3) -> (reference out=w10:refnum<k24>, "Stop"=w11:refnum<k24>)  [unwired: 2 in, 1 out]
  n222 = property class="AmateurStepperMotor"(reference=w10, "HoldOn"=FALSE) -> (reference out=w9:refnum<k24>)  [unwired: 1 in, 1 out]
  n223 = invoke class="AmateurStepperMotor" method="Dispose"(reference=w9) -> (error out=w6:errorcluster)  [unwired: 2 in, 2 out]
  n224 = invoke class="SerialPort" method="Close"(reference=w21, error in=w6) -> (reference out=w5:refnum<k24>, error out=w7:errorcluster)  [unwired: 1 in, 1 out]
  n225 = invoke class="Task" method="Wait"(reference=w11) -> ()  [unwired: 2 in, 3 out]
  n226 = Close Reference(reference=w5, error in (no error)=w7) -> (error out=w8:errorcluster)
  n227 = call <vilib>:"Simple Error Handler.vi"("error in (no error)"=w8) -> ()  [unwired: 1 in, 8 out]
  n228 = VISA Close(VISA resource name=w14, error in (no error)=w13) -> (error out=w23:errorcluster)
  n229 = call <instrlib>:"niDMM Close.vi"("error in (no error)"=w33, "instrument handle"=w34) -> ()  [unwired: 9 in, 1 out]
  n230 = call <instrlib>:"niDCPower Close.vi"("instrument handle"=w39) -> ()  [unwired: 10 in, 1 out]
  n231 = call "Ophir Error Message.vi"("error in (no error)"=w23) -> ()  [unwired: 3 in, 4 out]
